vi "PUT_send_key.vi"(8 "Cluster":T1, 10 "API Key":string="cheia04042025tema2restfulapi") -> (2 "body":string="{\n    \"message\": \"Did not attempt to load JSON data because the request Content-Type was not 'application/json'.\"\n}\n", 3 "headers":string="HTTP/1.1 415 UNSUPPORTED MEDIA TYPE\r\nServer: Werkzeug/3.1.3 Python/3.13.2\r\nDate: Thu, 27 Mar 2025 21:10:49 GMT\r\nContent-Type: application/json\r\nContent-Length: 116\r\nConnection: close\r\n\r\n")   [LabVIEW 2024]
uses:
  <vilib>/httpClient/PUTBuffer.vi
  <vilib>/httpClient/LabVIEWHTTPClient.lvlib
panel:
  out "JSON string":string="{\"security_access\":{\"auth_request\":true},\"key\":\"8978511683248979771\"}"
  out "error out json":errorcluster
  out "error out put":errorcluster
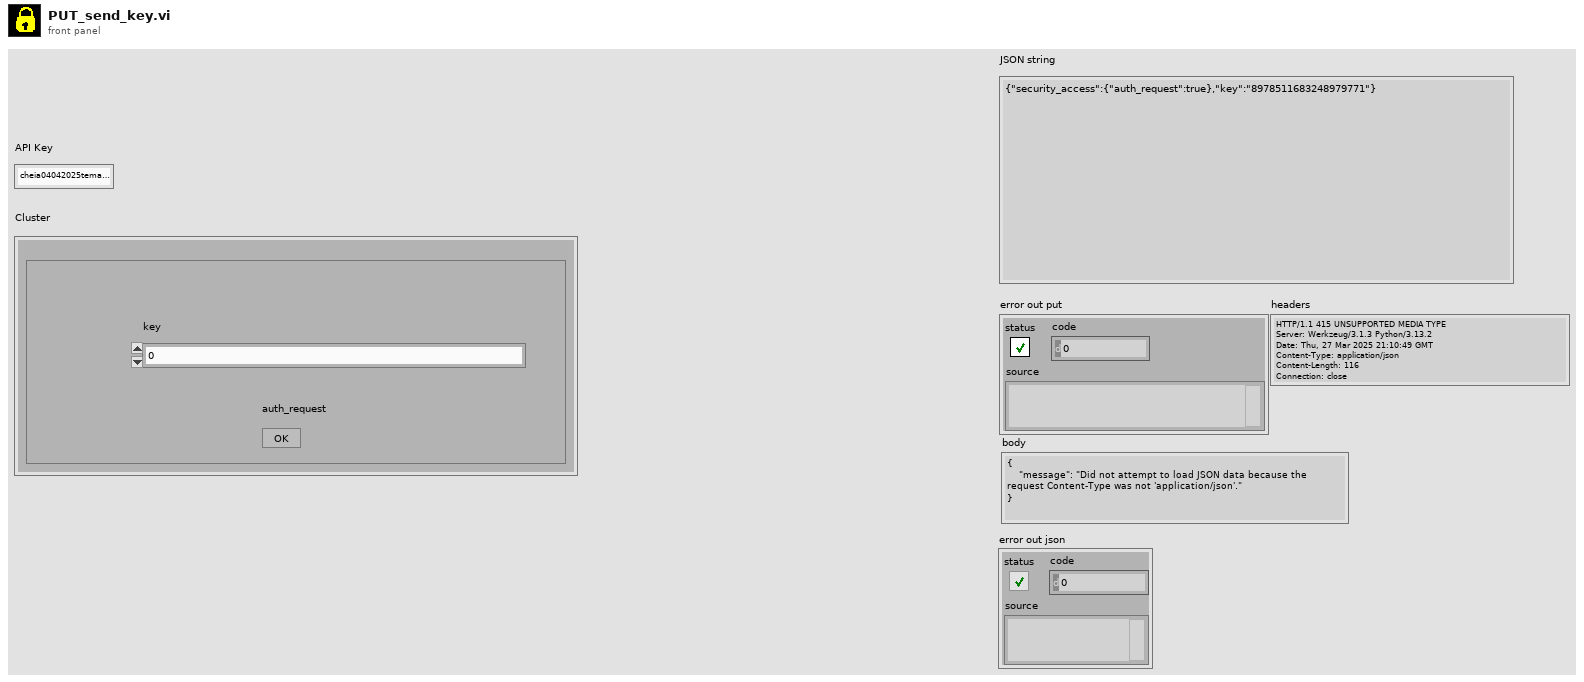
[diagram p1: front panel]
types:
  T1 = cluster{"security_access":cluster{"auth_request":bool, "key":u64}}
  T2 = typedef "LabVIEWHTTPClient.lvlib/ClientHandle.ctl" = refnum<k1>
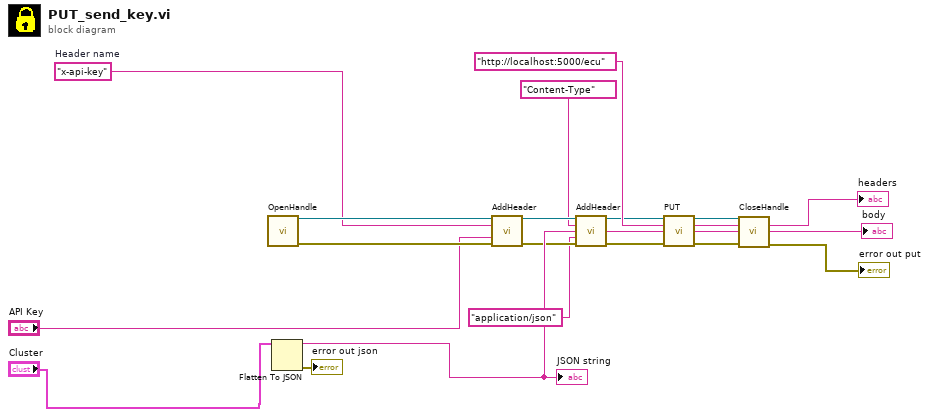
[diagram p0: block diagram]
diagram:
  w12 = "x-api-key"  # Header name
  n1 = call <vilib>:"OpenHandle.vi"() -> ("client handle out"=w13:T2, "error out"=w14:errorcluster)  [unwired: 14 in]
  n2 = Flatten To JSON(anything="Cluster") -> (JSON string=w8:string, 11:→"error out json":errorcluster)  [unwired: 2 in]
  "JSON string" <- w8
  n3 = call <vilib>:"AddHeader.vi"("client handle"=w13, "header"=w12, "value"="API Key", "error in (no error)"=w14) -> ("client handle out"=w6:T2, "error out"=w3:errorcluster)  [unwired: 10 in]
  n4 = call <vilib>:"AddHeader.vi"("client handle"=w6, "header"="Content-Type", "value"="application/json", "error in (no error)"=w3) -> ("client handle out"=w5:T2, "error out"=w4:errorcluster)  [unwired: 10 in]
  n5 = call-poly <vilib>:"PUT.vi"("client handle"=w5, "url"="http://localhost:5000/ecu", "buffer"=w8, "error in (no error)"=w4) -> ("client handle out"=w16:T2, "headers"=→"headers":string, "body"=→"body":string, "error out"=w15:errorcluster)  [unwired: 8 in]
  n6 = call <vilib>:"CloseHandle.vi"("client handle"=w16, "error in (no error)"=w15) -> ("error out"=→"error out put":errorcluster)  [unwired: 13 in]
